vi "PuTTY plink.vi"(8 "error in":errorcluster, 9 "working directory":path=path "", 10 "Hide DOS Window?":bool, 11 "Command(s) to Execute":string="{\"name\":\"buggyrun\"}\n{\t\"name\" : \"connect\"}\n{\t\"name\" : \"custom_cmd\"}\n{\t\"name\" : \"timeout\", \t\"timeout\" : 50000}\n{\"name\" : \"custom_cmd\"}\n{\"name\" : \"disconnect\"}\n{\"name\" : \"connect\"}\n{\"name\" : \"connect\"}\n{\t\"name\" : \"loadGel\", \"file\" : \"C:/Program Files/Texas Instruments/ccsv4/scripting/examples/TestServer/test.gel\"}\n{\"name\" : \"runGel\", \"expression\" : \"GEL_Reset()\"}\n{\"name\" : \"load\",\t\"program\" : \"Blink.out\"}\n{\t\"name\" : \"redirectCIO\",\t\"file\" : \"cio.txt\"}\n{\t\"name\" : \"setBreakpoint\",\t\"address\" : \"br1\"}\n\n") -> (0 "error out":errorcluster, 2 "Errors":string, 3 "Command Return Value(s)":string)   [LabVIEW 2018]
panel:
  out "Command Executed":string
  # "{\t\"name\" : \"connect\"}\n{\t\"name\" : \"timeout\", \t\"timeout\" : 50000}\n{\"name\" : \"load\",\t\"program\" : \"Blink.out\"}\n{\t\"name\" : \"setBreakpointAtLine\",\t\"file\":\"Blink.ino\", \"file2\":\"Blink.out\", \"line\": 50}"
  # "{\t\"name\" : \"setBreakpointAtLine\", \"address\":30,\"file\":\"Blink.cpp\"}"
  # "{\"name\":\"buggyrun\"}\n{\t\"name\" : \"connect\"}\n{\t\"name\" : \"custom_cmd\"}\n{\t\"name\" : \"timeout\", \t\"timeout\" : 50000}\n{\"name\" : \"custom_cmd\"}\n{\"name\" : \"disconnect\"}\n{\"name\" : \"connect\"}\n{\"name\" : \"connect\"}\n{\t\"name\" : \"loadGel\", \"file\" : \"C:/Program Files/Texas Instruments/ccsv4/scripting/examples/TestServer/test.gel\"}\n{\"name\" : \"runGel\", \"expression\" : \"GEL_Reset()\"}\n{\"name\" : \"load\",\t\"program\" : \"Blink.out\"}\n{\t\"name\" : \"redirectCIO\",\t\"file\" : \"cio.txt\"}\n{\t\"name\" : \"setBreakpoint\",\t\"address\" : \"SymbolDoesNotExist\"}\n{\t\"name\" : \"setBreakpoint\",\t\"address\" : \"main\"}\n{\t\"name\" : \"run\"}\n{\"name\" : \"redirectCIO\"}\n{\"name\" : \"runAsynch\",}\n{\t\"name\" : \"halt\"}\n{\t\"name\" : \"halt\"}\n\n{\t\"name\" : \"removeAllBreakpoints\"}\n{\t\"name\" : \"loadRawFromFile\",\t\"page\" : 0,\t\"address\" : 0x10000,\t\"file\" : \"loadRawFromFile.bin\",\t\"wordSize\" : 32,\t\"byteSwap\" : 0}\n{\t\"name\" : \"loadDataFromFile\",\t\"page\" : 0,\t\"address\" : 0x20000,\t\"file\" : \"loadDataFromFile.dat\",\t\"length\" : 1000}\n{\t\"name\" : \"loadRawFromFile\",\t\"page\" : 0,\t\"address\" : 0x10000,\t\"file\" : \"FileDoesNotExist.bin\",\t\"wordSize\" : 32,\t\"byteSwap\" : 0}\n{\t\"name\" : \"runGel\",\t\"expression\" : \"myTest()\"}\n{\t\"name\" : \"saveRawToFile\",\t\"page\" : 0,\t\"address\" : 0x10000,\t\"file\" : \"saveRawToFile.bin\",\t\"length\" : 1000,\t\"wordSize\" : 32,\t\"byteSwap\" : 0}\n{\t\"name\" : \"saveDataToFile\",\t\"page\" : 0,\t\"address\" : 0x20000,\t\"file\" : \"saveDataToFile.dat\",\t\"length\" : 1000,\t\"ioFormat\" : 1,\t\"append\" : 0}\n{\t\"name\" : \"writeData\",\t\"page\" : 0,\t\"address\" : 0x10000,\t\"value\" : 9,\t\t\"typeSize\" : 32};\n{\t\"name\" : \"readData\",\t\"page\" : 0,\t\"address\" : 0x10000,\t\"typeSize\" : 32,\t\"signed\" : 0}\n{\t\"name\" : \"readData\",\t\"page\" : 0,\t\"address\" : 0x10004,\t\"typeSize\" : 32,\t\"signed\" : 0}\n{\"name\" : \"stop\"}"
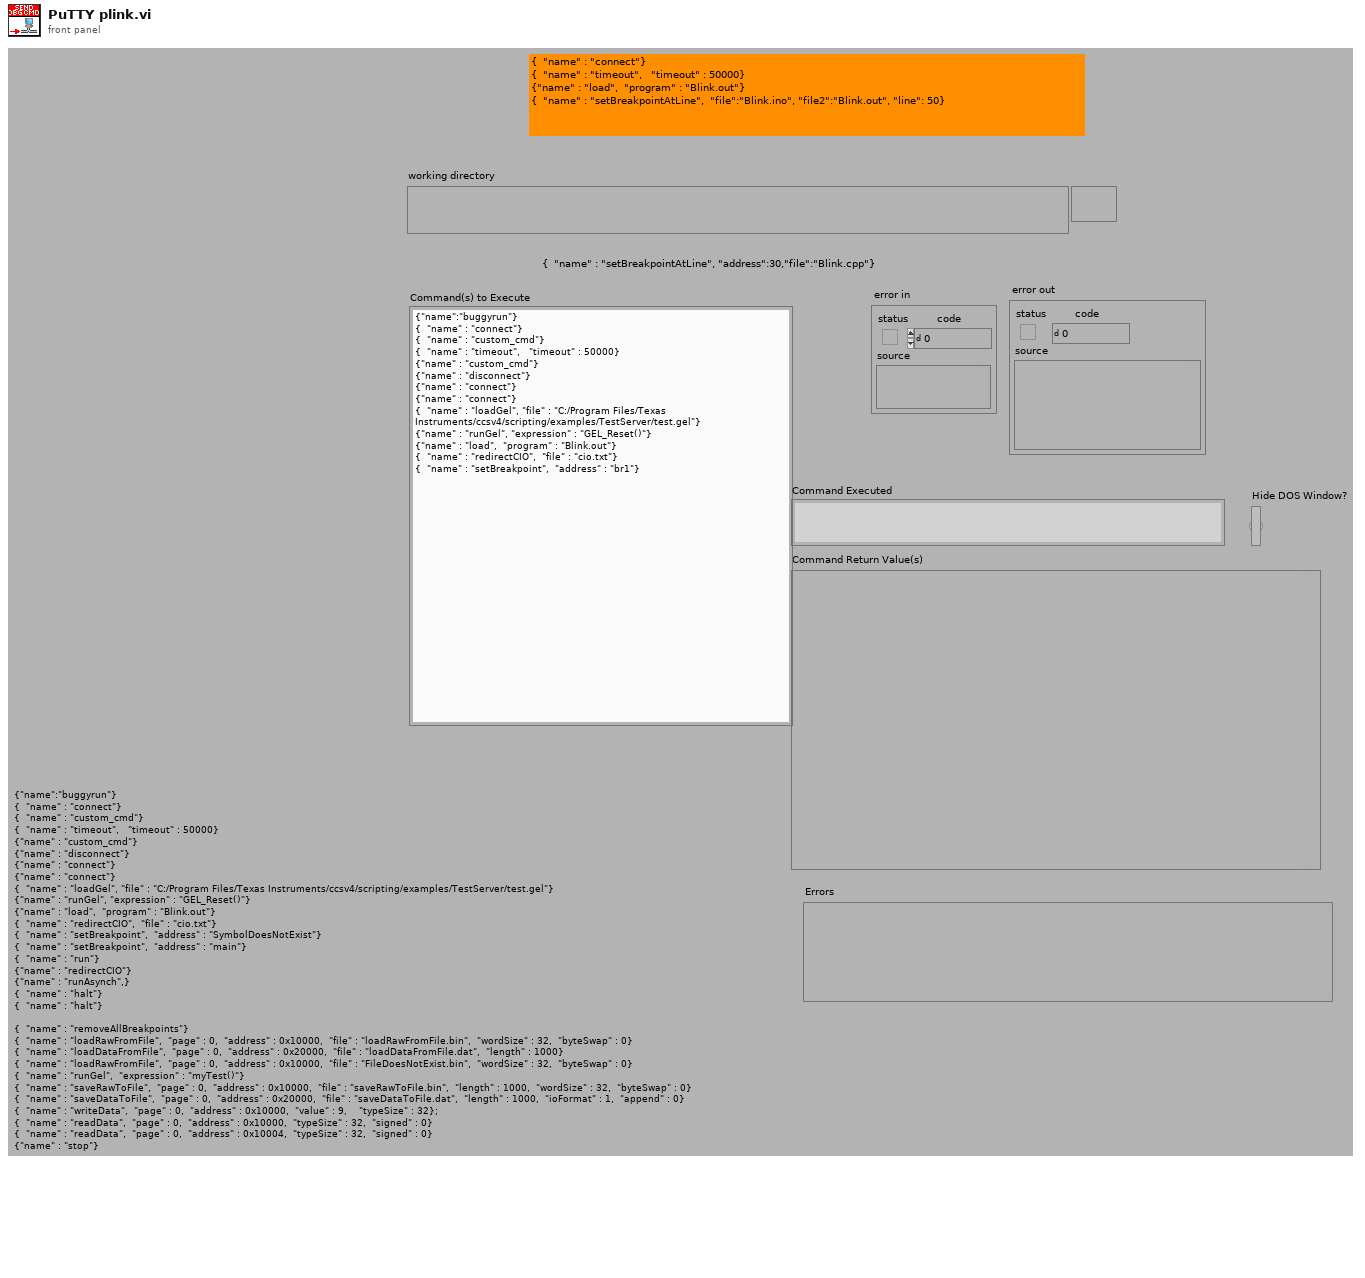
[diagram p1: front panel]
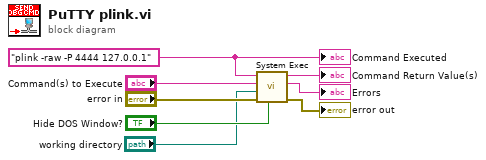
[diagram p0: block diagram]
diagram:
  w5 = "plink -raw -P 4444 127.0.0.1" ("format string")
  n1 = call <vilib>:"System Exec.vi"("run minimized? (F)"="Hide DOS Window?", "error in (no error)"="error in", "working directory"="working directory", "standard input"="Command(s) to Execute", "command line"=w5) -> ("error out"=→"error out":errorcluster, "standard error"=→"Errors":string, "standard output"=→"Command Return Value(s)":string)  [unwired: 1 in, 3 out]
  "Command Executed" <- w5
